vi "SaveDataToCSV2.vi"(4 "ReplaceFileName":string="_PTrack.csv", 6 "OmitFileName":string="_GFitPara", 7 "Header":string[](array[string]), 9 "Data":dbl[][](array[numeric]), 11 "パス":path) -> ()   [LabVIEW 2020]
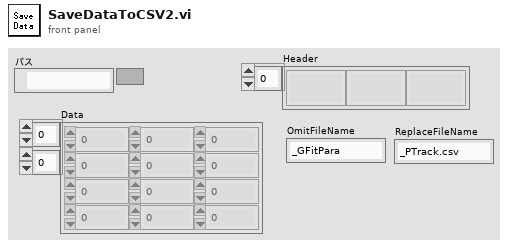
[diagram p1: front panel]
types:
  T1 = enum16{"open", "replace", "create", "open or create", "replace or create", "replace or create with confirmation"}
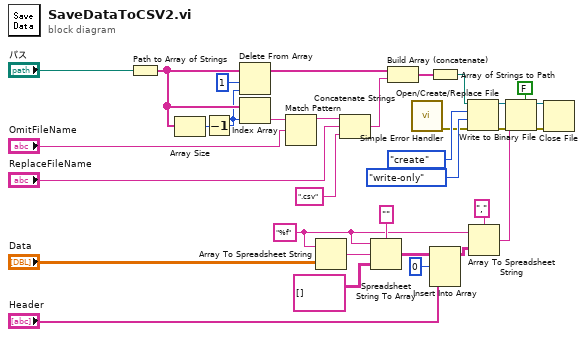
[diagram p0: block diagram]
diagram:
  w12 = "%f"
  n1 = Path to Array of Strings(0:"パス") -> (2:w20:string[])  [unwired: 1 out]
  n2 = Array Size(array=w20) -> (size(s)=w21:i32)
  n3 = Decrement(x=w21) -> (x-1=w8:i32)
  n4 = Delete From Array(array=w20, length=1 ("長さ"), index=w8) -> (array with subset deleted=w19:string[])  [unwired: 1 out]
  n5 = Index Array(array=w20, index=w8) -> (element=w7:string)
  n6 = Match Pattern(string=w7, regular expression="OmitFileName") -> (before substring=w5:string)  [unwired: 1 in, 3 out]
  n7 = Array To Spreadsheet String(array="Data", 3:w12) -> (spreadsheet string=w16:string)  [unwired: 1 out]
  n8 = Concatenate Strings(w5, "ReplaceFileName", ".csv" ("文字列")) -> (w32:string)
  n9 = Spreadsheet String To Array(delimiter (Tab)="" ("デリメタ(タブ)"), format string=w12, spreadsheet string=w16, array type (2D Dbl)=string[][] [] ("DataType")) -> (array=w10:string[][])
  n10 = Build Array (concatenate)(w19, w32) -> (w30:string[])
  n11 = Array of Strings to Path(0:w30) -> (2:w31:path)  [unwired: 1 out]
  n12 = Insert Into Array(array=w10, index (row)=0 ("指標 （行）"), new element="Header") -> (w14:string[][])  [unwired: 1 in]
  n13 = Open/Create/Replace File(file path (use dialog)=w31, operation (0:open)=T1."create" ("操作 (0:開く)"), access (0:read/write)=enum16{"read/write", "read-only", "write-only"}."write-only" ("アクセス （0:読み/書き）")) -> (refnum out=w27:refnum<file>)  [unwired: 1 in, 4 out]
  n14 = Array To Spreadsheet String(delimiter (Tab)="," ("デリミタ（タブ）"), array=w14, 3:w12) -> (spreadsheet string=w11:string)
  n15 = Write to Binary File ("Write File")(file (use dialog)=w27, data=w11, 5:FALSE ("配列または文字列サイズを先頭に追加?(T)")) -> (refnum out=w23:refnum<file>, error out=w24:errorcluster)  [unwired: 1 in, 3 out]
  n16 = Close File(refnum=w23, error in=w24) -> (error out=w25:errorcluster)  [unwired: 1 out]
  n17 = call <vilib>:"Simple Error Handler.vi"("error in (no error)"=w25) -> ()  [unwired: 1 in, 8 out]
